vi "Read sequences from disk.vi"(11 "error in (no error)":errorcluster) -> (15 "error out":errorcluster)   [LabVIEW 2011]
uses:
  Complete sequence cluster holder.ctl
  User input.ctl
  Sequence steps config..ctl
  Single criteria cluster.ctl
  Criteria types.ctl
  Boolean operation.ctl
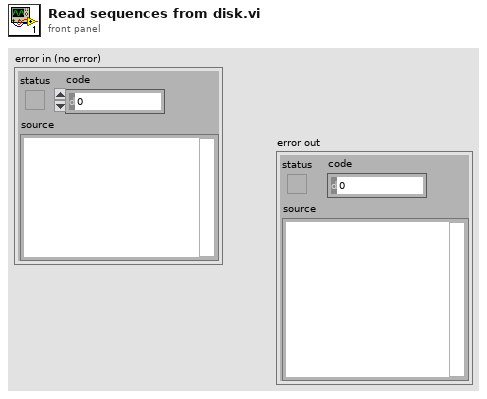
[diagram p1: front panel]
types:
  T1 = typedef "Complete sequence cluster holder.ctl" = cluster{"Sequence Name":string, "User input 1":T2, "Steps":T3[]}
  T2 = typedef "User input.ctl" = cluster{"Input name":string, "Minimum value ":dbl, "Maximum value":dbl, "Default value":dbl, "User inp enabled":bool}
  T3 = typedef "Sequence steps config..ctl" = cluster{"Enabled":bool, "Criteria 1":T4, "C1 op C2":T6, "Criteria 2":T4, "Action index":i32, "Action Name":string, "Action value":dbl}
  T4 = typedef "Single criteria cluster.ctl" = cluster{"Criteria":T5, "Time or analog value":dbl, "Primary IO index":i32, "Secondary  IO index":i32, "User_input":bool}
  T5 = typedef "Criteria types.ctl" = enum16{"No criteria(True)", "Time(s)", "Analog IO over", "Analog IO over or equal", "Analog IO under", "Analog IO under or equal", "Analog IO 1 minus Analog IO 2 over", "Digital IO True", "Digital IO False", "Operator approval"}
  T6 = typedef "Boolean operation.ctl" = enum16{"And", "Or", "Xor", "Nand", "Nor", "Nxor", "Implies"}
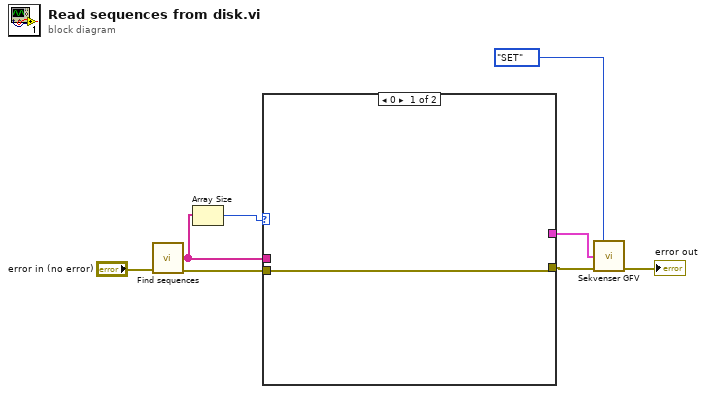
[diagram p0: block diagram]
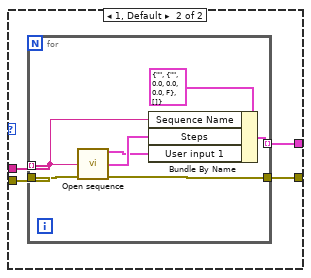
[diagram p2: hidden frame]
diagram:
  n1 = call "Find sequences.vi"("error in (no error)"="error in (no error)") -> ("Sequences"=w2:string[], "error out"=w4:errorcluster)  [unwired: 13 in]
  n2 = Array Size(array=w2) -> (size(s)=w1:i32)
  n3 = case shown="0" w1 {
    tunnel: [w9 w13] -> w5
    tunnel: w4 -> [w9 w12]
    tunnel: [_ w11] -> w3
    tunnel: w2 -> [_ w10]
    frame 0 {
    }
    frame 1, Default {
      n4 = for {
        tunnel: [w19] -> w13
        tunnel: w12 -> [w20]
        tunnel: w10 -> [w16] mode=indexing
        tunnel: [w15] -> w11 mode=indexing
        n5 = call "Open sequence.vi"("Sequence name"=w16, "error in (no error)"=w20) -> ("User input 1"=w14:T2, "Steps"=w17:T3[], "error out"=w19:errorcluster)  [unwired: 9 in, 2 out]
        n6 = Bundle By Name(cluster=T1 {"Sequence Name"="", "User input 1"={"Input name"="", "Minimum value "=0.0, "Maximum value"=0.0, "Default value"=0.0, "User inp enabled"=FALSE}, "Steps"=[]} ("Sequence in"), "Sequence Name"=w16, "Steps"=w17, "User input 1"=w14) -> (w15:T1)
      }
    }
  }
  n7 = call "Sekvenser GFV.vi"("Action(GET)"=enum16{"GET", "SET"}."SET", "Sequences"=w3, "error in (no error)"=w5) -> ("error out"=→"error out":errorcluster)  [unwired: 11 in, 1 out]
